vi "FieldControllerDemo.vi"() -> ()   [LabVIEW 2020]
uses:
  lib/SnapMB.lvlib
panel:
  out "Device 2 Error":string="No Error"
  out "Device 1 Error":string="No Error"
  out "RD Status":bool
  out "WR Status":bool
  in  "Ser Device ID":u8=2
  in  "Net Device ID":u8=1
  in  "Port":u16=502
  in  "Address":string="127.0.0.1"
  in  "Proto":i32(ring) items=["TCP", "UDP", "RTUOverTCP", "RTUOverUDP"]
  in  "Format":enum32{"RTU", "ASCII"}(ring)
  in  "Flow":enum32{"NONE", "RTS/CTS"}(ring)
  in  "Stop Bits":i32(ring)=1 items=["1"=1, "2"=2]
  in  "Data Bits":i32(ring)=8 items=["7"=7, "8"=8]
  in  "Parity":string(combo)="E"
  in  "ComPort":string(combo)="COM3"
  in  "Baudrate":i32(ring)=19200 items=["4800"=4800, "9600"=9600, "19200"=19200, "38400"=38400, "57600"=57600, "115200"=115200]
  in  "Scan Time (ms)":u32=500 min=10 step=1
  out "error out":errorcluster
  out "Run":bool
  in  "?":bool
  out "Total Job Time":i32
  in  "Amount":u16=16
  in  "Start":u16=17
  out "Data relayed":u16[](array[numeric])
  # "First Device (Read)"
  # "Second Device (Write)"
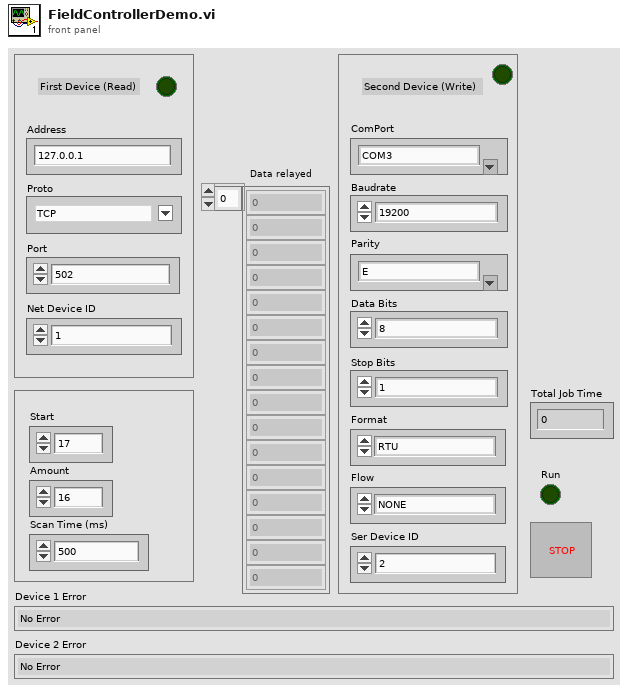
[diagram p1: front panel]
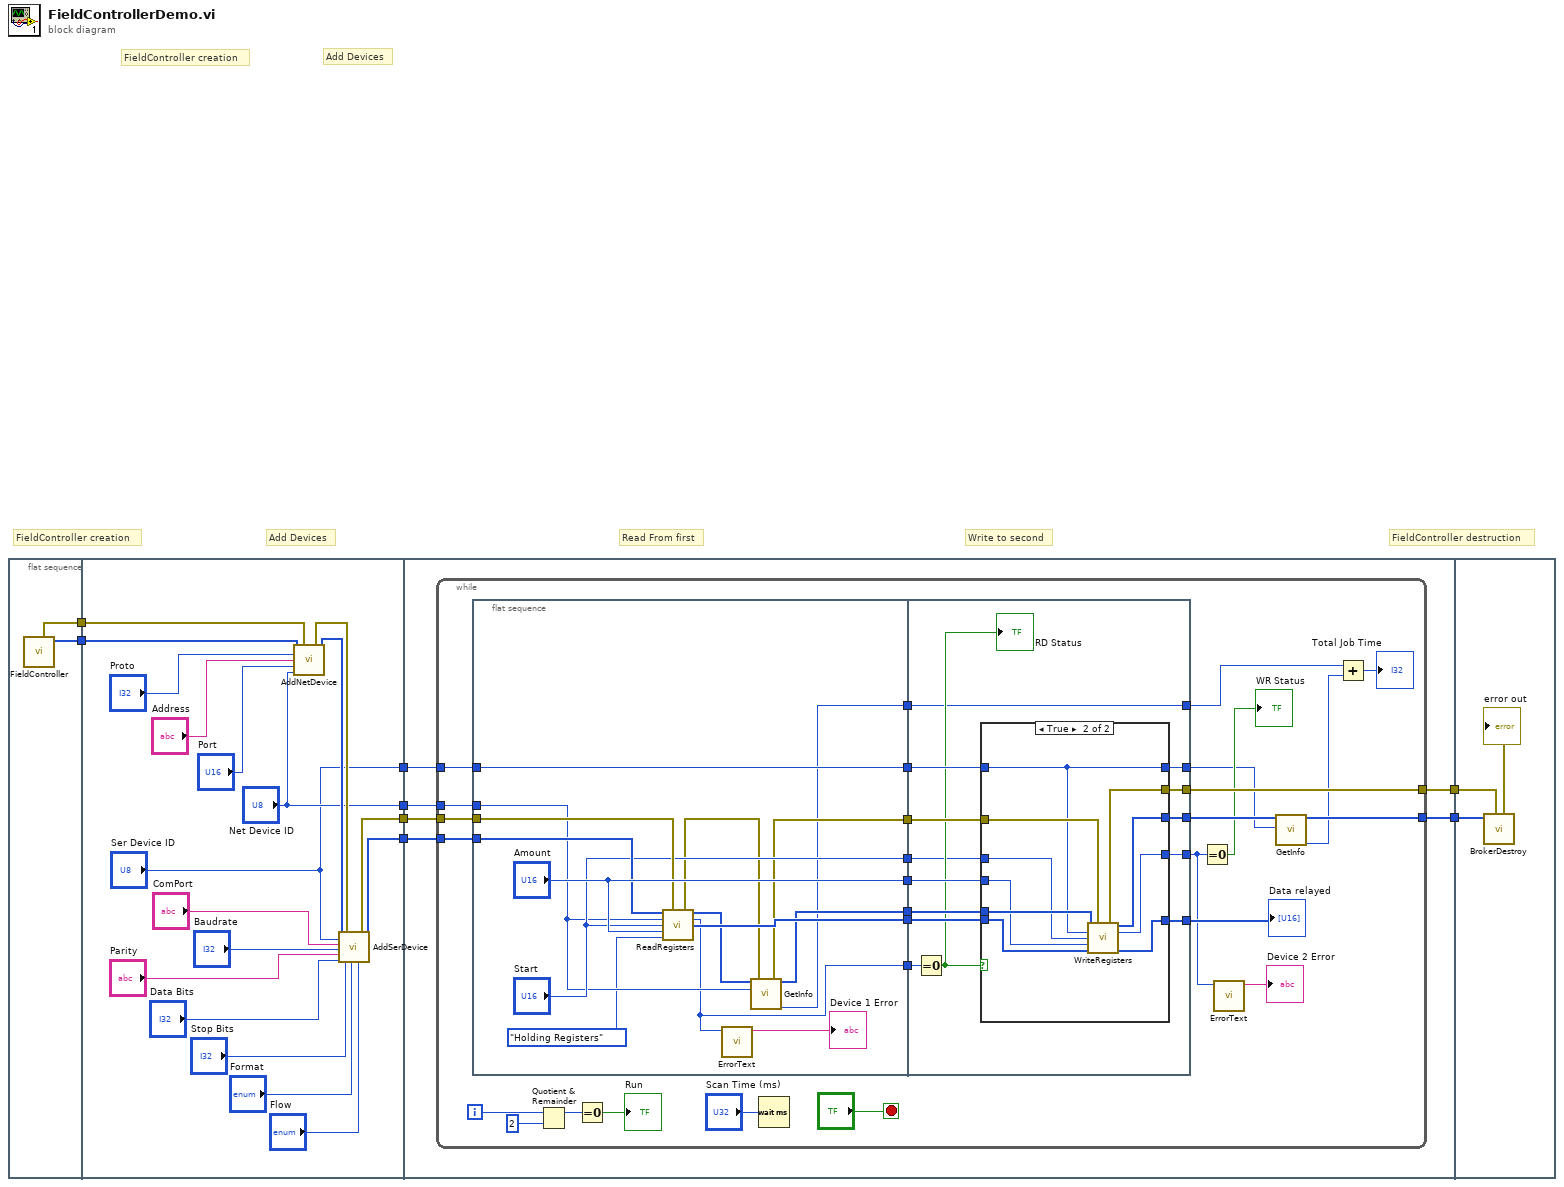
[diagram p0: block diagram]
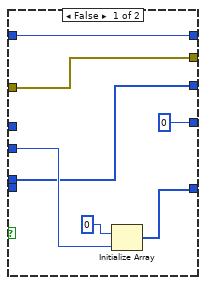
[diagram p2: hidden frame]
diagram:
  # "FieldController destruction"
  # "Write to second"
  # "Read From first"
  # "FieldController creation"
  # "Add Devices"
  # "FieldController creation"
  # "Add Devices"
  n1 = flat-sequence {
    tunnel: [w10] -> w8
    tunnel: [w9] -> w7
    tunnel: w8 -> [w16]
    tunnel: w7 -> [w15]
    tunnel: [w14] -> w4
    tunnel: [w13] -> w3
    tunnel: ["Net Device ID"] -> w2
    tunnel: ["Ser Device ID"] -> w1
    tunnel: [w32] -> w6
    tunnel: [w31] -> w5
    tunnel: w1 -> [w29]
    tunnel: w2 -> [w30]
    tunnel: w3 -> [w33]
    tunnel: w4 -> [w34]
    tunnel: w6 -> [w112]
    tunnel: w5 -> [w111]
    frame #0 {
      n2 = call "FieldController.vi"() -> ("Field Controller"=w10:u64[], "error out"=w9:errorcluster)  [unwired: 10 in]
    }
    frame #1 {
      n3 = call "AddNetDevice.vi"("Handle In"=w16, "error in"=w15, "Proto"="Proto", "Address"="Address", "Port"="Port", "Device ID"="Net Device ID") -> ("error out"=w24:errorcluster, "Handle Out"=w25:u64[])  [unwired: 7 in, 1 out]
      n4 = call "AddSerDevice.vi"("Handle In"=w25, "Device ID"="Ser Device ID", "Port"="ComPort", "Baudrate"="Baudrate", "Parity"="Parity", "Data Bits"="Data Bits", "error in (no error)"=w24, "Stop Bits"="Stop Bits", "Format"="Format", "Flow"="Flow") -> ("error out"=w13:errorcluster, "Handle Out"=w14:u64[])  [unwired: 7 in, 1 out]
    }
    frame #2 {
      n5 = while {
        tunnel: w34 -> [w52]
        tunnel: w33 -> [w51]
        tunnel: [w50] -> w32
        tunnel: [w49] -> w31
        tunnel: w30 -> [w48]
        tunnel: w29 -> [w46]
        i -> [w53]
        stop <- "?" stop-if-true
        n6 = flat-sequence {
          tunnel: [w78] -> w63
          tunnel: ["Amount"] -> w62
          tunnel: [w65] -> w61
          tunnel: w52 -> [w76]
          tunnel: w51 -> [w75]
          tunnel: w48 -> [w68]
          tunnel: [w74] -> w47
          tunnel: w46 -> [w74]
          tunnel: ["Start"] -> w44
          tunnel: [w72] -> w43
          tunnel: [w70] -> w42
          tunnel: [w67] -> w41
          tunnel: w63 -> [w91]
          tunnel: w62 -> [w90]
          tunnel: w61 -> [w88]
          tunnel: [w87] -> w59
          tunnel: [w86] -> w36
          tunnel: [w85] -> w49
          tunnel: [w84] -> w58
          tunnel: w47 -> [w83]
          tunnel: w44 -> [w81]
          tunnel: w43 -> [w92]
          tunnel: w42 -> [w89]
          tunnel: [w80] -> w39
          tunnel: w41 -> [w80]
          tunnel: [w79] -> w37
          frame #0 {
            n7 = call "ReadRegisters.vi"("Handle In"=w76, "error in (no error)"=w75, "Device ID"=w68, "Read Start"="Start", "Read Amount"="Amount", "Area"=enum16{"Holding Registers", "Input Registers"}."Holding Registers") -> ("error out"=w69:errorcluster, "Handle Out"=w71:u64[], "Result"=w65:i32, "RD Data"=w78:u16[])  [unwired: 6 in]
            n8 = call "ErrorText.vi"("ErrNo"=w65) -> ("ErrMessage"=→"Device 1 Error":string)  [unwired: 9 in, 1 out]
            n9 = call "GetInfo.vi"("Broker In"=w71, "DeviceID"=w68, "error in"=w69) -> ("error out"=w70:errorcluster, "Broker Out"=w72:u64[], "JobTime"=w67:i32)  [unwired: 10 in, 4 out]
          }
          frame #1 {
            n10 = Equal To 0?(x=w88) -> (x = 0?=w82:bool)
            "RD Status" <- w82
            n11 = case shown="True" w82 {
              tunnel: w92 -> [w94 w109]
              tunnel: w91 -> [_ w108]
              tunnel: w90 -> [w97 w107]
              tunnel: w89 -> [w95 w106]
              tunnel: [w98 w101] -> w87
              tunnel: [0 ("Result") w100] -> w86
              tunnel: [w95 w105] -> w85
              tunnel: [w94 w104] -> w84
              tunnel: w83 -> [w93 w102]
              tunnel: w81 -> [_ w103]
              tunnel: [w93 w102] -> w79
              frame False {
                n12 = Initialize Array(u16 0 ("element"), w97) -> (w98:u16[])
              }
              frame True {
                n13 = call "WriteRegisters.vi"("Handle In"=w109, "error in (no error)"=w106, "Device ID"=w102, "Write Start"=w103, "Write Amount"=w107, "WR Data"=w108) -> ("error out"=w105:errorcluster, "Handle Out"=w104:u64[], "Result"=w100:i32, "Data Written"=w101:u16[])  [unwired: 6 in]
              }
            }
          }
        }
        n14 = Quotient & Remainder(x=w53, y=2) -> (x-y*floor(x/y)=w56:i32)  [unwired: 1 out]
        n15 = Equal To 0?(x=w56) -> (x = 0?=→"Run":bool)
        n16 = Wait (ms)(milliseconds to wait="Scan Time (ms)") -> ()  [unwired: 1 out]
        n17 = Equal To 0?(x=w36) -> (x = 0?=→"WR Status":bool)
        n18 = call "ErrorText.vi"("ErrNo"=w36) -> ("ErrMessage"=→"Device 2 Error":string)  [unwired: 9 in, 1 out]
        n19 = call "GetInfo.vi"("Broker In"=w58, "DeviceID"=w37) -> ("Broker Out"=w50:u64[], "JobTime"=w38:i32)  [unwired: 11 in, 5 out]
        n20 = Add(x=w39, y=w38) -> (x+y=→"Total Job Time":i32)
        "Data relayed" <- w59
      }
    }
    frame #3 {
      n21 = call "BrokerDestroy.vi"("error in (no error)"=w111, "Handle In"=w112) -> ("error out"=→"error out":errorcluster)  [unwired: 9 in]
    }
  }
